vi "addTemperatureFrame.vi"(8 "error in (no error)":errorcluster, 9 "TriggerIRQ":bool, 10 "WaitForTrigger":bool, 11 "Subnet in":refnum<class "Subnet.lvclass">) -> (0 "error out":errorcluster, 3 "Subnet out":refnum<class "Subnet.lvclass">)   [LabVIEW 2016, in "Subnet.lvclass"]
uses:
  Subnet.lvclass
  Subnet.lvclass/Subnet.ctl
  Common_RT_Modbus/IModbus/IModbus.lvclass
  Common_RT_MTILC/MTILC/MTILC.lvclass
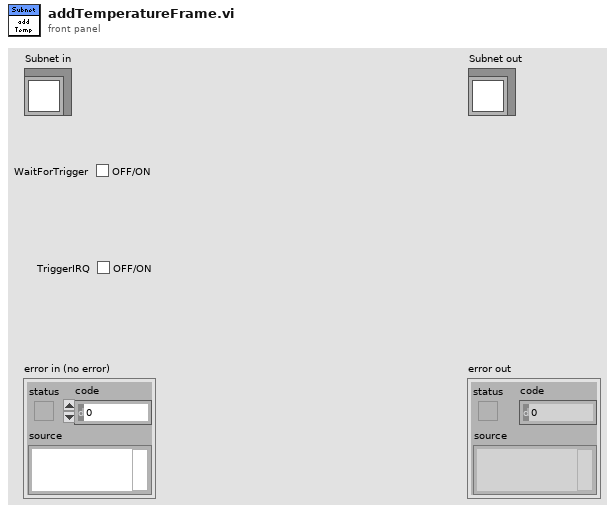
[diagram p1: front panel]
types:
  T1 = typedef "RTModbus.lvlib/TxFrame.ctl" = cluster{"Data":u8[], "WaitForTrigger":bool, "WaitForRx":u16, "TriggerIRQ":bool, "DelayMicroseconds":u16, "DelayMilliseconds":u16, "Timestamp":bool}
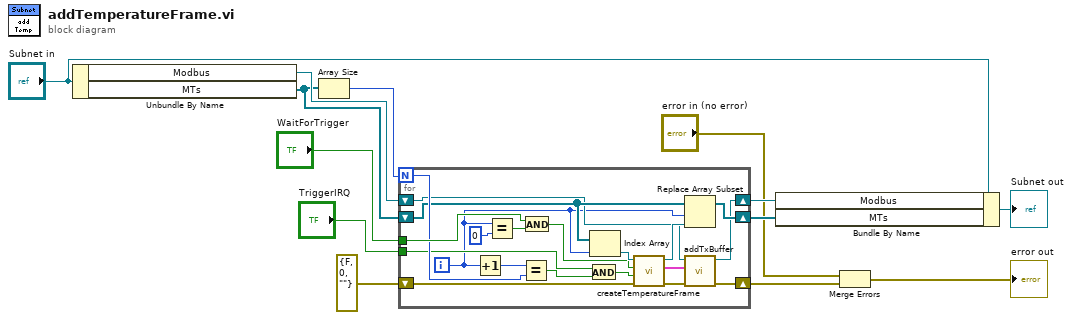
[diagram p0: block diagram]
diagram:
  n1 = Unbundle By Name("Subnet in") -> ("Modbus"=w13:refnum<class "IModbus.lvclass">, "MTs"=w11:refnum<class "MTILC.lvclass">[])
  n2 = Array Size(array=w11) -> (size(s)=w10:i32)
  n3 = for {
    N: w10 -> [w27]
    shift-right: [w19] -> w5
    shift-left: w13 -> [w21]
    shift-right: [w22] -> w4
    shift-left: w11 -> [w23]
    tunnel: "WaitForTrigger" -> [w32]
    tunnel: "TriggerIRQ" -> [w25]
    shift-right: [w16] -> w3
    shift-left: errorcluster {"status"=FALSE, "code"=0, "source"=""} ("error out") -> [w17]
    i -> [w15]
    n4 = Increment(x=w15) -> (x+1=w14:i32)
    n5 = Equal?(x=w15, y=0) -> (x = y?=w33:bool)
    n6 = Equal?(x=w14, y=w27) -> (x = y?=w28:bool)
    n7 = And(x=w32, y=w33) -> (x .and. y?=w29:bool)
    n8 = And(x=w25, y=w28) -> (x .and. y?=w26:bool)
    n9 = Index Array(array=w23, index=w15) -> (element=w30:refnum<class "MTILC.lvclass">)
    n10 = call "createTemperatureFrame.vi"("error in (no error)"=w17, "TriggerIRQ"=w26, "WaitForTrigger"=w29, "MTILC in"=w30) -> ("error out"=w18:errorcluster, "TxFrame"=w20:T1, "MTILC out"=w24:refnum<class "MTILC.lvclass">)  [unwired: 5 in]
    n11 = Replace Array Subset(array=w23, new element=w24, index=w15) -> (w22:refnum<class "MTILC.lvclass">[])
    n12 = call-dynamic "addTxBuffer.vi"("error in (no error)"=w18, "TxFrame"=w20, "IModbus in"=w21) -> ("error out"=w16:errorcluster, "IModbus out"=w19:refnum<class "IModbus.lvclass">)  [unwired: 7 in]
  }
  n13 = Bundle By Name(cluster="Subnet in", "Modbus"=w5, "MTs"=w4) -> (→"Subnet out":refnum<class "Subnet.lvclass">)
  n14 = Merge Errors("error in (no error)", w3) -> (→"error out":errorcluster)
